vi "Validate_command.vi"(8 "error in (no error)":errorcluster, 11 "ZMQ multipart message in":string[](array[string])) -> (0 "error out":errorcluster, 2 "Valid?":bool, 3 "ZMQ multipart message out":string[](array[string]))   [LabVIEW 2019, in "Service.lvlib"]
uses:
  Service.lvlib
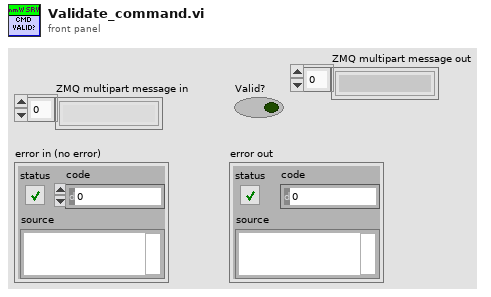
[diagram p1: front panel]
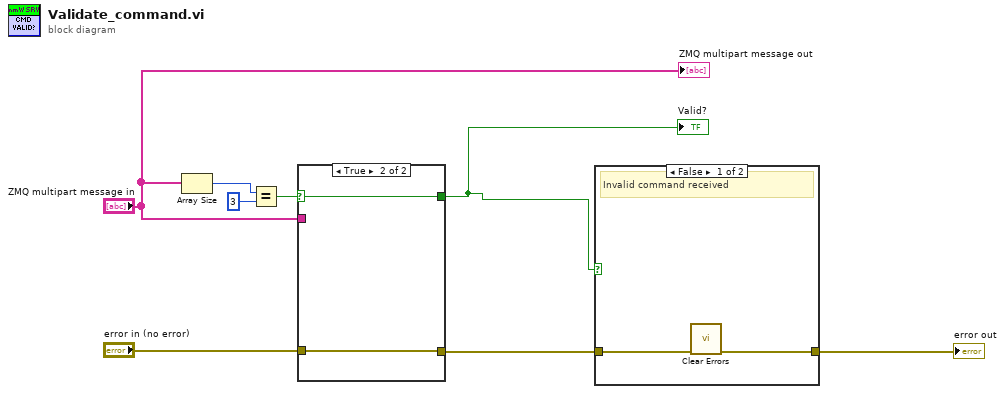
[diagram p0: block diagram]
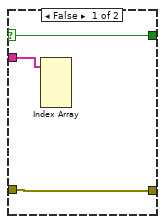
[diagram p3: hidden frame]
diagram:
  n1 = Array Size(array="ZMQ multipart message in") -> (size(s)=w4:i32)
  n2 = Equal?(x=w4, y=3) -> (x = y?=w6:bool)
  n3 = case shown="True" w6 {
    selector: w6 -> [w11 w13]
    tunnel: [w11 w13] -> w3
    tunnel: "ZMQ multipart message in" -> [w10 _]
    tunnel: "error in (no error)" -> [w9 w12]
    tunnel: [w9 w12] -> w2
    frame False {
      n4 = Index Array(array=w10) -> ()  [unwired: 4 in, 4 out]
    }
    frame True {
    }
  }
  "Valid?" <- w3
  n5 = case shown="False" w3 {
    tunnel: w2 -> [w15 w16]
    tunnel: [w14 w16] -> w1
    frame False {
      # "Invalid command received"
      n6 = call <vilib>:"Clear Errors.vi"("error in (no error)"=w15) -> ("error out"=w14:errorcluster)  [unwired: 5 in, 1 out]
    }
    frame True {
    }
  }
  "error out" <- w1
  "ZMQ multipart message out" <- "ZMQ multipart message in"
